vi "Obtain_Variable_Value.vi"(7 "path":string[][](array[string]), 8 "index":i32, 10 "JSON result":string="{\"result\":[[\"Position\",\"Speed\",\"Control\",\"error DAQ\",\"tiempo\",\"spPos\",\"spVel\",\"is late?\"],[9.99,0.000000,0.000000,\"Unsupported type of variable\",0.000000,0.000000,0.000000,false]]}") -> (3 "currentValue":dbl=9.99)   [LabVIEW 2020]
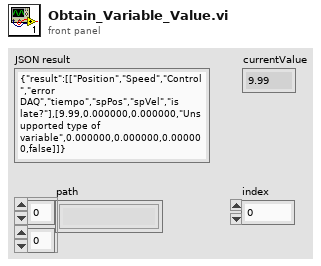
[diagram p1: front panel]
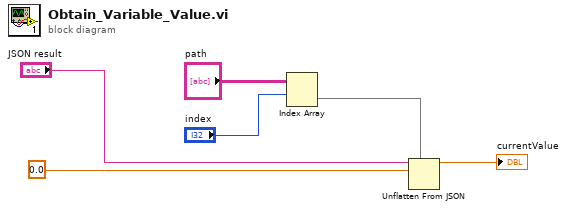
[diagram p0: block diagram]
diagram:
  n1 = Index Array(array="path", index (row)="index") -> (element=w2:string[])  [unwired: 1 in]
  n2 = Unflatten From JSON(path=w2, JSON string="JSON result", type and defaults=0.0 ("Numeric")) -> (value=→"currentValue":dbl)  [unwired: 4 in, 1 out]
